vi "EventUser.vi"(8 "error in (no error)":errorcluster) -> (0 "error out":errorcluster, 2 "Menue":refnum<user-event>)   [LabVIEW 2016, in "MenueItem.lvclass"]
uses:
  MenueItem.lvclass
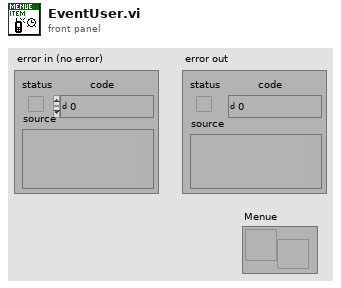
[diagram p1: front panel]
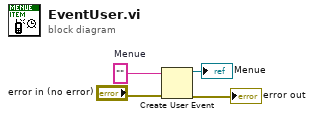
[diagram p0: block diagram]
diagram:
  w4 = ""  # Menue
  n1 = Create User Event(user event datatype=w4, error in="error in (no error)") -> (user event=→"Menue":refnum<user-event>, error out=→"error out":errorcluster)
